vi "Flow Imform.vi"() -> ()   [LabVIEW 2019]
uses:
  Main Process Class VI/Ctrl/Flow Action Name.ctl
panel:
  in  "Flow Act Ref":refnum<vi>
  in  "Robot Imform Board Out":bool
  in  "Imform Robot board In":bool
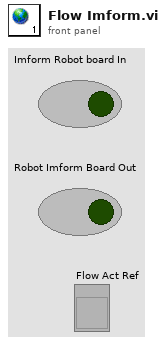
[diagram p1: front panel]
diagram:
